vi "Read Name.vi"(3 "((Pointer))":refnum<class "((Pointer)).lvclass">) -> (1 "Name Out":string)   [LabVIEW 2016, in "((Pointer)).lvclass"]
uses:
  ((Pointer)).lvclass
  ((Pointer)).lvclass/((Pointer)).ctl
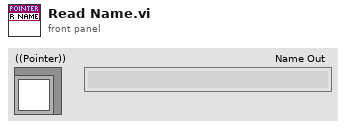
[diagram p1: front panel]
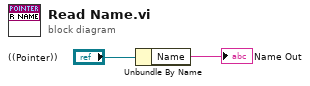
[diagram p0: block diagram]
diagram:
  n1 = Unbundle By Name("((Pointer))") -> ("Name"=→"Name Out":string)
